vi "Import CSV.vi"(8 "error in (no error)":errorcluster, 11 "Controller in":refnum<class "Controller.lvclass">) -> (0 "error out":errorcluster, 3 "Controller out":refnum<class "Controller.lvclass">)   [LabVIEW 2013, in "SET Project Editor.lvlib" / "Controller.lvclass"]
uses:
  Controller.lvclass
  Controller.lvclass/Controller.ctl
  SET Project Data/Project Data Class/Project Data.lvclass
  <vilib>/ActorFramework/Message Enqueuer/Message Enqueuer.lvclass/Message Enqueuer.ctl
  <vilib>/ActorFramework/Message Enqueuer/Enqueue.vi
  <vilib>/ActorFramework/Message Priority Queue/Priority Enqueue.vi
  SET Project Data/Resource Data Class/Resource Data.lvclass
  UI View Messages/UI Refresh Data Msg/UI Refresh Data Msg.lvclass
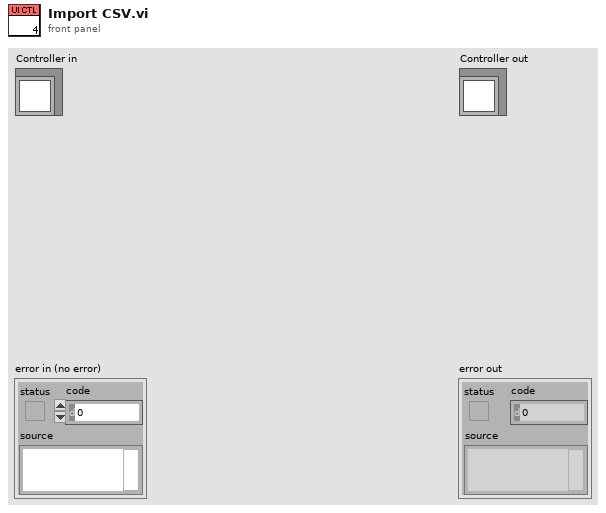
[diagram p1: front panel]
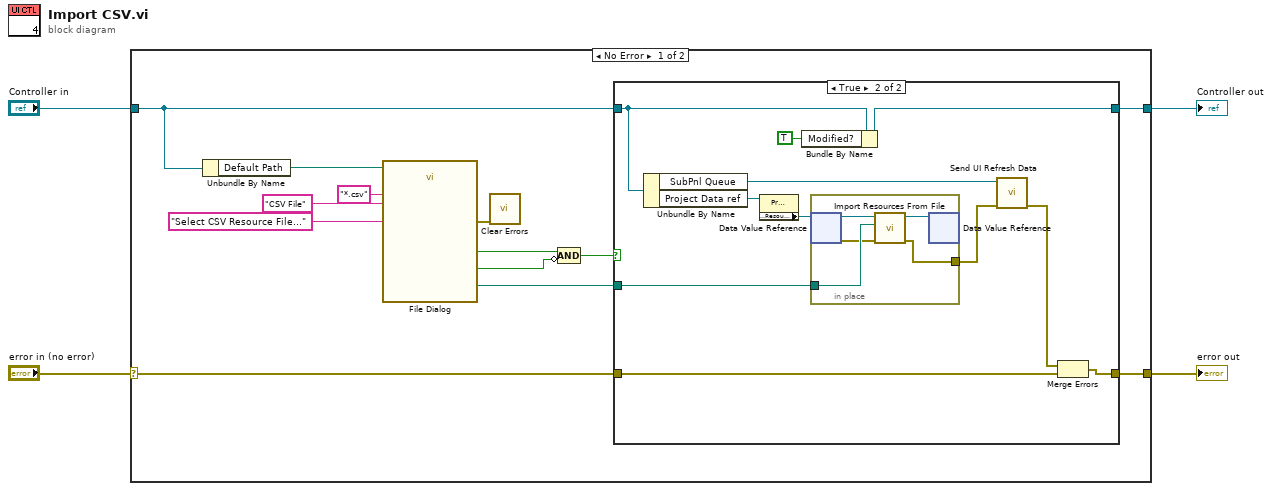
[diagram p0: block diagram]
diagram:
  n1 = case shown="No Error" "error in (no error)" {
    selector: "error in (no error)" -> [w5 w37]
    tunnel: [w6 w37] -> w3
    tunnel: [w7 w36] -> w1
    tunnel: "Controller in" -> [w9 w36]
    frame No Error {
      n2 = Unbundle By Name(w9) -> ("Default Path"=w16:path)
      n3 = call "File Dialog"("start path"=w16, "prompt"="Select CSV Resource File...", "pattern (all files)"="*.csv", "pattern label"="CSV File") -> ("selected path"=w8:path, "exists"=w13:bool, "cancelled"=w14:bool, "error out"=w15:errorcluster)  [unwired: 8 in]
      n4 = call <vilib>:"Clear Errors.vi"("error in (no error)"=w15) -> ()  [unwired: 6 in, 1 out]
      n5 = Compound Arithmetic op=AND(w13, invert w14) -> (w10:bool)
      n6 = case shown="True" w10 {
        tunnel: w9 -> [w19 w25]
        tunnel: w8 -> [_ w30]
        tunnel: [w19 w24] -> w7
        tunnel: [w18 w26] -> w6
        tunnel: w5 -> [w18 w27]
        frame False {
        }
        frame True {
          n7 = Unbundle By Name(w25) -> ("SubPnl Queue"=w22:refnum<class "Message Enqueuer.lvclass">, "Project Data ref"=w29:refnum<data-value>)
          n8 = property class="Project Data.lvclass"(reference=w29) -> ("Properties:Resource Data ref"=w28:refnum<data-value>)  [unwired: 1 in, 2 out]
          n9 = Bundle By Name(cluster=w25, "Modified?"=TRUE) -> (w24:refnum<class "Controller.lvclass">)
          n10 = in-place {
            in-place-border: w30 -> [w35]
            in-place-border: [w31] -> w20
            n11 = in-place-dvr #1(w28) -> (w34:refnum<class "Resource Data.lvclass">, w33:errorcluster)
            n12 = call "Import Resources From File.vi"("error in (no error)"=w33, "file path (use dialog)"=w35, "LangFile.lvclass in"=w34) -> ("error out"=w31:errorcluster, "LangFile.lvclass out"=w32:refnum<class "Resource Data.lvclass">)  [unwired: 7 in]
            n13 = in-place-dvr #1(w32) -> ()  [unwired: 2 out]
          }
          n14 = call "Send UI Refresh Data.vi"("error in (no error)"=w20, "Message Enqueuer"=w22) -> ("error out"=w21:errorcluster)  [unwired: 8 in, 1 out]
          n15 = Merge Errors(w21, w27) -> (w26:errorcluster)
        }
      }
    }
    frame Error {
    }
  }
  "error out" <- w3
  "Controller out" <- w1
